vi "RESTful Build INI File.vi"(0 "target reference":refnum<vi>, 1 "RESTful VI service information":T5, 5 "VI Configurations":T9[](array[typedef]), 7 "data.Privilege Mapping":T1(array[cluster]), 9 "Routing Templates":T2[](array[typedef]), 11 "error in (no error)":errorcluster, 12 "buildContext":refnum<vi>, 14 "relative VI paths":path[](array[path])) -> (3 "AMQP INI":path, 4 "dup target reference":refnum<vi>, 6 "INI filepath":path, 8 "AMQP XML":path, 10 "XML filepath":path, 15 "error out":errorcluster)   [LabVIEW 2020]
uses:
  <vilib>/AppBuilder/AB_Classes/Source/RESTfulVI/Configure_RESTfulVI/AB_RESTful_Configuration.ctl
  <vilib>/AppBuilder/AB_Classes/Source/RESTfulVI/Configure_RESTfulVI/AB_RESTful_VIType.ctl
  <vilib>/AppBuilder/AB_Classes/Source/RESTfulVI/Configure_RESTfulVI/AB_RESTful_OutputType.ctl
  <vilib>/AppBuilder/AB_Classes/Source/RESTfulVI/Configure_RESTfulVI/AB_RESTful_OutputFormat.ctl
  <vilib>/AppBuilder/Engine/RESTful INI Generator/AB_RESTful_ServiceInfo.ctl
  <vilib>/AppBuilder/AB_Classes/RESTful/AB_RESTful_ServiceAttribute.ctl
  <vilib>/AppBuilder/AB_Classes/RESTful/AB_RESTful_ServiceAttributeType.ctl
  <vilib>/AppBuilder/Engine/RESTful INI Generator/AB_RESTful_ServiceType.ctl
  <vilib>/AppBuilder/AB_Classes/RESTful/AB_RESTful_RoutingTemplate.ctl
  <vilib>/AppBuilder/AB_Classes/RESTful/AB_RESTful_RoutingType.ctl
  <vilib>/AppBuilder/AB_Classes/RESTful/AB_RESTful_HTTPMethodType.ctl
  <vilib>/AppBuilder/Engine/WebServiceDescription/Web Service Description Info.ctl
  <vilib>/AppBuilder/Engine/WebServiceDescription/Response.ctl
  <vilib>/AppBuilder/Engine/WebServiceDescription/Terminal Info.ctl
  <vilib>/AppBuilder/Engine/WebServiceDescription/LVDataTypes/LVType/LVType.lvclass
  <vilib>/AppBuilder/Engine/WebServiceDescription/URL Mapping Info.ctl
  <vilib>/AppBuilder/Engine/WebServiceDescription/Web Service Description.lvlib
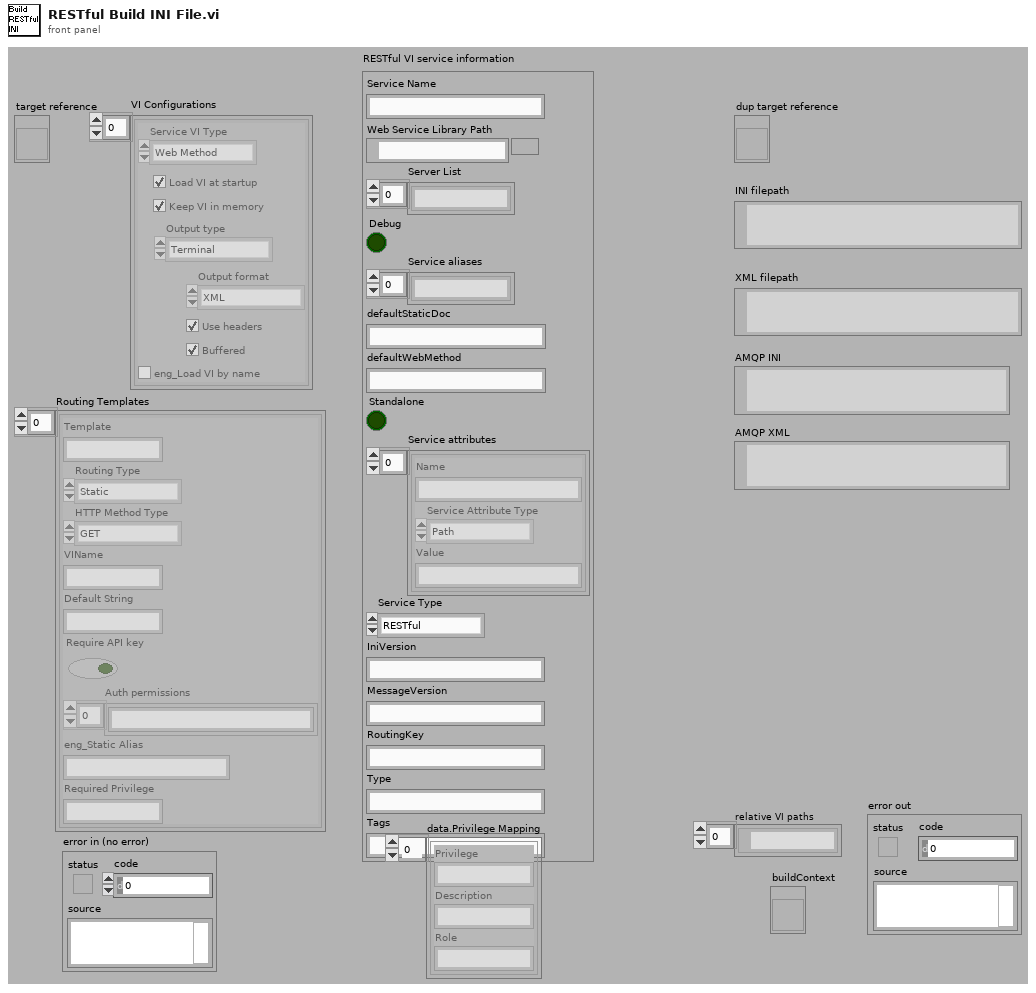
[diagram p1: front panel]
types:
  T1 = cluster{"Privilege":string, "Description":string, "Role":string}[]
  T2 = typedef "AB_RESTful_RoutingTemplate.ctl" = cluster{"Template":string, "Routing Type":T3, "HTTP Method Type":T4, "VIName":string, "Default String":string, "Require API key":bool, "Auth permissions":string[], "eng_Static Alias":string, "Required Privilege":string}
  T3 = typedef "AB_RESTful_RoutingType.ctl" = enum32{"Method", "Static"}
  T4 = typedef "AB_RESTful_HTTPMethodType.ctl" = enum32{"GET", "POST", "PUT", "DELETE"}
  T5 = typedef "AB_RESTful_ServiceInfo.ctl" = cluster{"Service Name":string, "Web Service Library Path":path, "Server List":string[], "Debug":bool, "Service aliases":string[], "defaultStaticDoc":string, "defaultWebMethod":string, "Standalone":bool, "Service attributes":T6[], "Service Type":T8, "IniVersion":string, "MessageVersion":string, "RoutingKey":string, "Type":string, "Tags":string}
  T6 = typedef "AB_RESTful_ServiceAttribute.ctl" = cluster{"Name":string, "Service Attribute Type":T7, "Value":string}
  T7 = typedef "AB_RESTful_ServiceAttributeType.ctl" = enum32{"String", "Path"}
  T8 = typedef "AB_RESTful_ServiceType.ctl" = enum32{"RESTful", "SOAP", "AMQP"}
  T9 = typedef "AB_RESTful_Configuration.ctl" = cluster{"Service VI Type":T10, "Load VI at statup":bool, "Keep VI in memory":bool, "Output type":T11, "Output format":T12, "Use headers":bool, "Buffered":bool, "eng_Load VI by name":bool}
  T10 = typedef "AB_RESTful_VIType.ctl" = enum32{"Web Method", "Auxiliary", "eng_Internal", "eng_Content"}
  T11 = typedef "AB_RESTful_OutputType.ctl" = enum32{"Terminal", "Stream"}
  T12 = typedef "AB_RESTful_OutputFormat.ctl" = enum32{"XML", "Text", "HTML", "JSON"}
  T13 = typedef "Web Service Description.lvlib/Web Service Description Info.ctl" = cluster{"Web Service Name":string, "Responses":T14[], "Mappings":T16[]}
  T14 = typedef "Web Service Description.lvlib/Response.ctl" = cluster{"VI Name":string, "Output format":T12, "Output type":T11, "Outputs":T15[]}
  T15 = typedef "Web Service Description.lvlib/Terminal Info.ctl" = cluster{"Name":string, "Type":refnum<class "LVType.lvclass">}
  T16 = typedef "Web Service Description.lvlib/URL Mapping Info.ctl" = cluster{"Mapping String":string, "HTTP Method Type":T4, "Require API Key":bool, "Inputs":T15[], "VI Name":string, "Require Authentication":bool}
  T17 = enum16{"open", "replace", "create", "open or create", "replace or create", "replace or create with confirmation"}
  T18 = cluster{"Controls for XML":T15[], "Indicators for XML":T15[]}
  T19 = typedef "RESTful VI Terminal Info Summary.ctl" = cluster{"escaped terminal name":string, "conn pane number":i32, "control type":string, "indicator?":bool, "unescaped terminal name":string, "element list":string, "dimensions":u32, "YArrayType":string, "element owner type":string, "class instantiation VI":string}
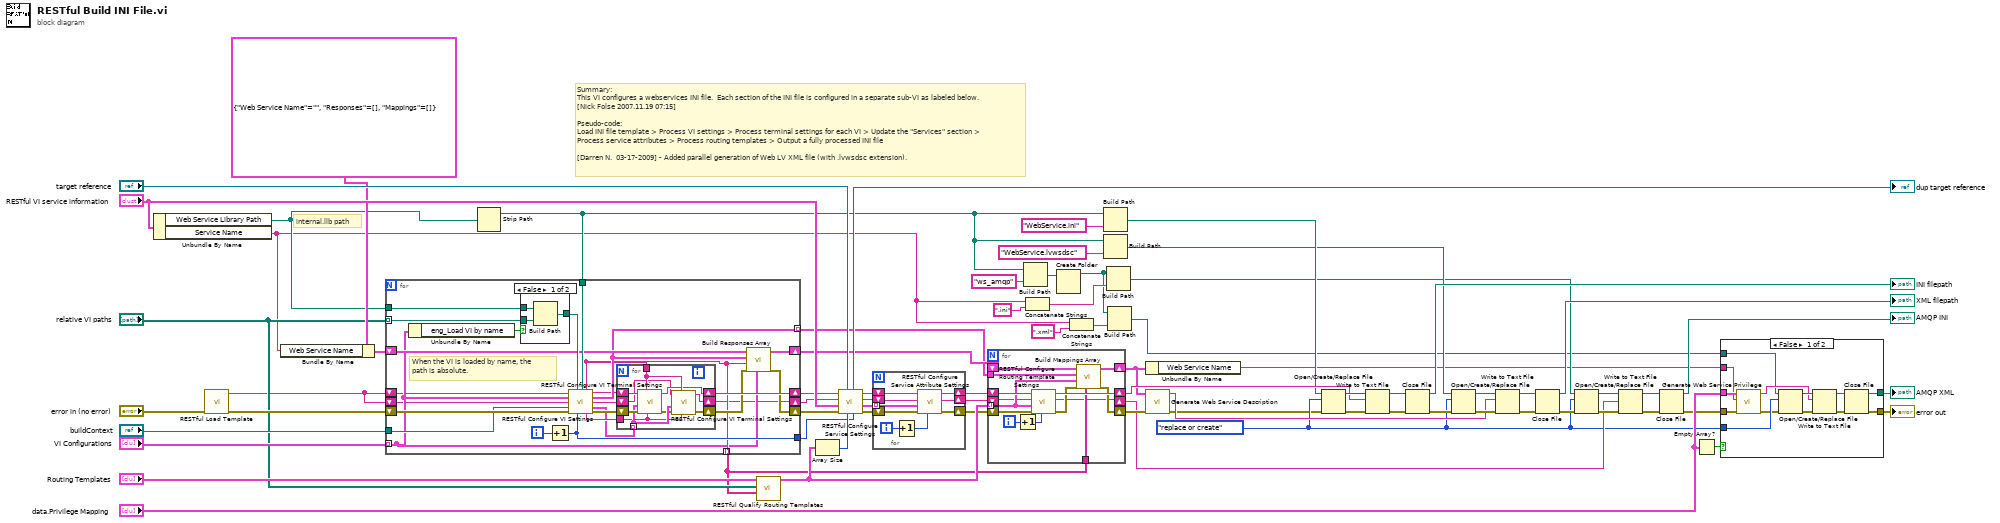
[diagram p0: block diagram]
diagram:
  w4 = T17."replace or create" ("operation (0:open)")
  # "internal.llb path"
  # "Summary: \nThis VI configures a webservices INI file.  Each section of the INI file is configured in a separate sub-VI as labeled below.\n[Nick Folse 2007.11.19 07:15]\n\nPseudo-code:\nLoad INI file template > Process VI settings > Process terminal settings for each VI > Update the \"Services\" section > Process service attributes > Process routing templates > Output a fully processed INI file\n\n[Darren N.  03-17-2009] - Added parallel generation of Web LV XML file (with .lvwsdsc extension)."
  n1 = Unbundle By Name("RESTful VI service information") -> ("Web Service Library Path"=w34:path, "Service Name"=w11:string)
  n2 = call <vilib>:"RESTful Load Template.vi"("error in (no error)"="error in (no error)") -> ("error out"=w74:errorcluster, "INI File Template"=w26:string)  [unwired: 9 out]
  n3 = Bundle By Name(cluster=T13 {"Web Service Name"="", "Responses"=[], "Mappings"=[]} ("Description"), "Web Service Name"=w11) -> (w49:T13)
  n4 = Strip Path(path=w34) -> (stripped path=w14:path)  [unwired: 1 out]
  n5 = for {
    tunnel: "VI Configurations" -> [w82] mode=indexing
    shift-right: [w97] -> w27
    shift-left: w26 -> [w79]
    shift-right: [w90] -> w44
    shift-left: w74 -> [w99]
    tunnel: w34 -> [w94]
    tunnel: "buildContext" -> [w86]
    tunnel: w14 -> [w93]
    shift-right: [w89] -> w47
    shift-left: w49 -> [w92]
    tunnel: [w88] -> w45 mode=indexing
    tunnel: "relative VI paths" -> [w87] mode=indexing
    tunnel: [w84] -> w28
    tunnel: [w83] -> w40 mode=indexing
    shift-right: [w77] -> w25
    shift-left: w26 -> [w78]
    i -> [w85]
    # "When the VI is loaded by name, the\npath is absolute."
    n6 = Unbundle By Name(w82) -> ("eng_Load VI by name"=w81:bool)
    n7 = case shown="False" w81 {
      tunnel: [w102 w103] -> w95
      tunnel: w94 -> [w101 _]
      tunnel: w87 -> [w100 w103]
      frame False {
        n8 = Build Path(base path=w101, name or relative path=w100) -> (appended path=w102:path)
      }
      frame True {
      }
    }
    n9 = Increment(x=w85) -> (x+1=w84:i32)
    n10 = call <vilib>:"RESTful Configure VI Settings.vi"("Master Text In"=w79, "vi path"=w95, "base path"=w93, "RESTful VI configuration"=w82, "AMQP Ini In"=w78, "buildContext"=w86, "error in"=w99, "VI Number (1..N)"=w84) -> ("qualified VI name"=w83:string, "Master Text Out"=w76:string, "Controls and Indicators for XML"=w88:T18, "AMQP Ini Out"=w75:string, "Terminal Info Summary"=w80:T19[], "VI_Section_Heading"=w96:string, "error out"=w98:errorcluster)  [unwired: 1 in]
    n11 = for {
      tunnel: w96 -> [w111]
      shift-right: [w109] -> w91
      shift-left: w98 -> [w113]
      shift-right: [w106] -> w97
      shift-left: w76 -> [w107]
      tunnel: w80 -> [w112] mode=indexing
      tunnel: w83 -> [w108]
      shift-right: [w104] -> w77
      shift-left: w75 -> [w105]
      n12 = call <vilib>:"RESTful Configure VI Terminal Settings.vi"("VI Section Heading"=w111, "VI Name"=w108, "error in"=w113, "Terminal Info Summary"=w112, "Master Text In"=w107) -> ("error out"=w110:errorcluster, "Master Text Out"=w106:string)  [unwired: 2 in, 3 out]
      n13 = call <vilib>:"RESTful Configure VI Terminal Settings.vi"("VI Section Heading"=w111, "VI Name"=w108, "error in"=w110, "Terminal Info Summary"=w112, "Master Text In"=w105) -> ("error out"=w109:errorcluster, "Master Text Out"=w104:string)  [unwired: 2 in, 3 out]
    }
    n14 = call <vilib>:"Build Responses Array.vi"("RESTful VI configuration"=w82, "error in (no error)"=w91, "VI Name"=w83, "Controls and Indicators for XML"=w88, "Description in"=w92) -> ("error out"=w90:errorcluster, "Description out"=w89:T13)  [unwired: 5 in]
  }
  n15 = call <vilib>:"RESTful Qualify Routing Templates.vi"("qualified VI names"=w40, "relative VI paths"="relative VI paths", "Routing Templates"="Routing Templates") -> ("Routing Templates out"=w43:T2[])  [unwired: 8 in]
  n16 = Array Size(array=w43) -> (size(s)=w71:i32)
  n17 = call <vilib>:"RESTful Configure Service Settings.vi"("Number VIs"=w28, "Number of Routing Templates"=w71, "target reference"="target reference", "error in"=w44, "RESTful VI service information"="RESTful VI service information", "AMQP Ini In"=w25, "Master Text In"=w27) -> ("error out"=w37:errorcluster, "Service attributes"=w35:T6[], "AMQP Ini Out"=w24:string, "Master Text Out"=w39:string, "dup target reference"=→"dup target reference":refnum<vi>)
  n18 = for {
    shift-right: [w120] -> w38
    shift-left: w39 -> [w121]
    shift-right: [w119] -> w36
    shift-left: w37 -> [w118]
    tunnel: w35 -> [w116] mode=indexing
    shift-right: [w114] -> w23
    shift-left: w24 -> [w115]
    i -> [w122]
    n19 = Increment(x=w122) -> (x+1=w117:i32)
    n20 = call <vilib>:"RESTful Configure Service Attribute Settings.vi"("Service Attribute Number (1..N)"=w117, "error in"=w118, "RESTful service attribute"=w116, "AMQP Ini In"=w115, "Master Text In"=w121) -> ("error out"=w119:errorcluster, "AMQP Ini Out"=w114:string, "Master Text Out"=w120:string)  [unwired: 4 in]
  }
  n21 = for {
    shift-right: [w128] -> w48
    shift-left: w36 -> [w135]
    shift-right: [w134] -> w65
    shift-left: w38 -> [w136]
    tunnel: w43 -> [w127] mode=indexing
    shift-right: [w131] -> w10
    shift-left: w47 -> [w130]
    tunnel: w45 -> [w126]
    tunnel: w40 -> [w125]
    shift-right: [w123] -> w22
    shift-left: w23 -> [w124]
    i -> [w132]
    n22 = Increment(x=w132) -> (x+1=w133:i32)
    n23 = call <vilib>:"RESTful Configure Routing Template Settings.vi"("Routing Template Number (1..N)"=w133, "error in"=w135, "RESTful VI routing template"=w127, "AMQP Ini In"=w124, "Master Text In"=w136) -> ("error out"=w129:errorcluster, "AMQP Ini Out"=w123:string, "Master Text Out"=w134:string)  [unwired: 4 out]
    n24 = call <vilib>:"Build Mappings Array.vi"("VI Names"=w125, "error in (no error)"=w129, "RESTful VI routing template"=w127, "Controls and Indicators for XML"=w126, "Description in"=w130) -> ("error out"=w128:errorcluster, "Description out"=w131:T13)  [unwired: 5 in]
  }
  n25 = Build Path(base path=w14, name or relative path="ws_amqp") -> (appended path=w15:path)
  n26 = Concatenate Strings(w11, ".ini" ("string")) -> (w19:string)
  n27 = Create Folder(path (use dialog)=w15) -> (created path=w16:path)  [unwired: 2 in, 2 out]
  n28 = Concatenate Strings(w11, ".xml" ("string")) -> (w17:string)
  n29 = Build Path(base path=w14, name or relative path="WebService.lvwsdsc" ("format string")) -> (appended path=w52:path)
  n30 = Build Path(base path=w14, name or relative path="WebService.ini" ("format string")) -> (appended path=w63:path)
  n31 = Build Path(base path=w16, name or relative path=w19) -> (appended path=w20:path)
  n32 = Build Path(base path=w16, name or relative path=w17) -> (appended path=w6:path)
  n33 = Unbundle By Name(w10) -> ("Web Service Name"=w7:string)
  n34 = call <vilib>:"Generate Web Service Description.vi"("error in (no error)"=w48, "Description"=w10) -> ("error out"=w3:errorcluster, "Web Service Description String"=w46:string)  [unwired: 8 out]
  n35 = Open/Create/Replace File(file path (use dialog)=w63, error in=w3, operation (0:open)=w4) -> (refnum out=w68:refnum<file>, error out=w66:errorcluster)  [unwired: 4 out]
  n36 = Write to Text File(file (use dialog)=w68, text=w65, error in=w66) -> (refnum out=w69:refnum<file>, error out=w67:errorcluster)  [unwired: 2 out]
  n37 = Close File(refnum=w69, error in=w67) -> (path=→"INI filepath":path, error out=w53:errorcluster)
  n38 = Open/Create/Replace File(file path (use dialog)=w52, error in=w53, operation (0:open)=w4) -> (refnum out=w54:refnum<file>, error out=w57:errorcluster)  [unwired: 1 in, 3 out]
  n39 = Write to Text File(file (use dialog)=w54, text=w46, error in=w57) -> (refnum out=w55:refnum<file>, error out=w56:errorcluster)  [unwired: 2 out]
  n40 = Close File(refnum=w55, error in=w56) -> (path=→"XML filepath":path, error out=w29:errorcluster)
  n41 = Open/Create/Replace File(file path (use dialog)=w20, error in=w29, operation (0:open)=w4) -> (refnum out=w33:refnum<file>, error out=w30:errorcluster)  [unwired: 1 in, 3 out]
  n42 = Write to Text File(file (use dialog)=w33, text=w22, error in=w30) -> (refnum out=w32:refnum<file>, error out=w31:errorcluster)  [unwired: 2 out]
  n43 = Close File(refnum=w32, error in=w31) -> (path=→"AMQP INI":path, error out=w2:errorcluster)
  n44 = Empty Array?(array="data.Privilege Mapping") -> (empty?=w9:bool)
  n45 = case shown="False" w9 {
    tunnel: "data.Privilege Mapping" -> [w145 _]
    tunnel: w7 -> [w143 _]
    tunnel: w6 -> [w142 _]
    tunnel: [w141 _] -> w5
    tunnel: w4 -> [w140 _]
    tunnel: [w138 w150] -> w1
    tunnel: w2 -> [w137 w150]
    frame False {
      n46 = call <vilib>:"Generate Web Service Privilege.vi"("error in (no error)"=w137, "Service Name"=w143, "data.Privilege Mapping"=w145) -> ("error out"=w139:errorcluster, "resulting string"=w144:string)  [unwired: 7 in]
      n47 = Open/Create/Replace File(file path (use dialog)=w142, error in=w139, operation (0:open)=w140) -> (refnum out=w148:refnum<file>, error out=w146:errorcluster)  [unwired: 1 in, 3 out]
      n48 = Write to Text File(file (use dialog)=w148, text=w144, error in=w146) -> (refnum out=w149:refnum<file>, error out=w147:errorcluster)  [unwired: 2 out]
      n49 = Close File(refnum=w149, error in=w147) -> (path=w141:path, error out=w138:errorcluster)
    }
    frame True {
    }
  }
  "error out" <- w1
  "AMQP XML" <- w5
